vi "Set Start Trigger (Analog Edge).vi"(5 "Retriggerable (F)":bool, 7 "Pre-Trigger Duration (0 s)":dbl, 8 "error in (no error)":errorcluster, 9 "Trigger Channel":string, 10 "Analog Edge Condition":T1, 11 "Data Logging Specification Ref in":T3) -> (0 "error out":errorcluster, 3 "Data Logging Specification Ref out":T3)   [LabVIEW 2020, in "NI_VS Data Logging API.lvlib"]
doc: "Specifies a trigger condition on which to start logging data. You also can specify whether to log channel data immediately preceding the trigger condition and whether logging is retriggerable, meaning the data logging session watches for subsequent occurrences of the start trigger after the first logging operation finishes. By default, logging stops after one operation.\n\nYou must manually select the polymorphic instance to use."
uses:
  <vilib>/NI VeriStand/Execution/DataLogging/NI_VS Data Logging API.lvlib
  <vilib>/NI VeriStand/Execution/DataLogging/DataLoggingSpecification Ref.ctl
  NationalInstruments.VeriStand.ClientAPI
  <vilib>/NI VeriStand/Execution/DataLogging/Analog Edge Condition.ctl
  <vilib>/NI VeriStand/Execution/DataLogging/Slope.ctl
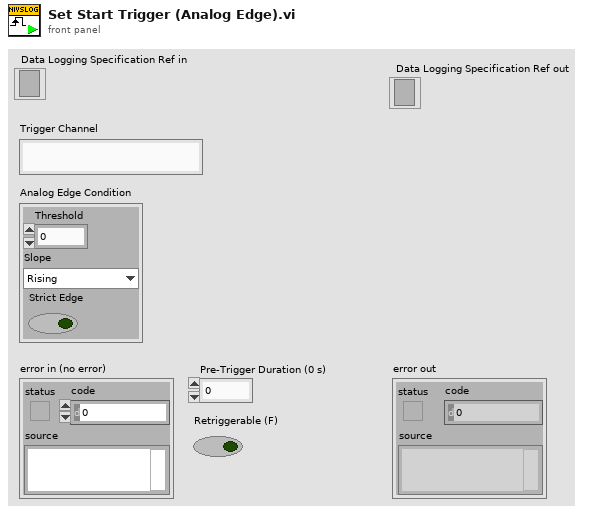
[diagram p1: front panel]
types:
  T1 = typedef "NI_VS Data Logging API.lvlib/Analog Edge Condition.ctl" = cluster{"Threshold":dbl, "Slope":T2, "Strict Edge":bool}
  T2 = typedef "NI_VS Data Logging API.lvlib/Slope.ctl" = enum16{"Rising", "Falling"}
  T3 = typedef "NI_VS Data Logging API.lvlib/DataLoggingSpecification Ref.ctl" = refnum<k24>
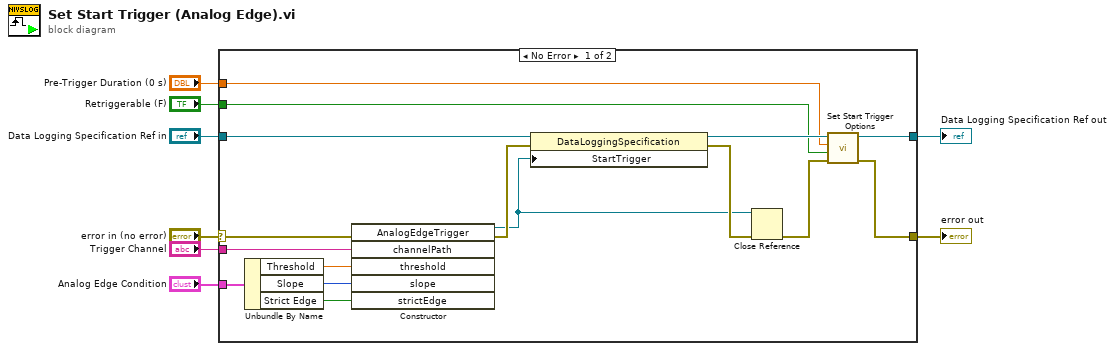
[diagram p0: block diagram]
diagram:
  n1 = case shown="No Error" "error in (no error)" {
    selector: "error in (no error)" -> [w17 w26]
    tunnel: "Trigger Channel" -> [w16 _]
    tunnel: "Data Logging Specification Ref in" -> [w22 w25]
    tunnel: [w19 w25] -> w6
    tunnel: [w18 w26] -> w5
    tunnel: "Analog Edge Condition" -> [w14 _]
    tunnel: "Pre-Trigger Duration (0 s)" -> [w10 _]
    tunnel: "Retriggerable (F)" -> [w9 _]
    frame No Error {
      n2 = Unbundle By Name(w14) -> ("Threshold"=w13:dbl, "Slope"=w12:T2, "Strict Edge"=w11:bool)
      n3 = constructor class="AnalogEdgeTrigger"(error in=w17, "channelPath"=w16, "threshold"=w13, "slope"=w12, "strictEdge"=w11) -> (reference out=w15:refnum<k24>, error out=w24:errorcluster)  [unwired: 2 in, 5 out]
      n4 = property class="DataLoggingSpecification"(reference=w22, error in=w24, "StartTrigger"=w15) -> (reference out=w21:T3, error out=w23:errorcluster)
      n5 = Close Reference(reference=w15, error in (no error)=w23) -> (error out=w20:errorcluster)
      n6 = call <vilib>:"Set Start Trigger Options.vi"("error in (no error)"=w20, "Retriggerable"=w9, "Pre-Trigger Duration"=w10, "Data Logging Specification Ref in"=w21) -> ("error out"=w18:errorcluster, "Data Logging Specification Ref out"=w19:T3)  [unwired: 6 in]
    }
    frame Error {
    }
  }
  "error out" <- w5
  "Data Logging Specification Ref out" <- w6
